vi "Subscribe to Results.vi"(8 "error in (no error)":errorcluster, 10 "Result Observer":refnum<class "Result Observer.lvclass">, 11 "LUnit Test Case V2 In":refnum<class "LUnit Test Case V2.lvclass">) -> (0 "error out":errorcluster, 3 "LUnit Test Case V2 Out":refnum<class "LUnit Test Case V2.lvclass">)   [LabVIEW 2020, in "LUnit Test Case V2.lvclass"]
uses:
  LUnit Test Case V2.lvclass
  Result Observer/Result Observer.lvclass
  LUnit Test Case V2.lvclass/LUnit Test Case V2.ctl
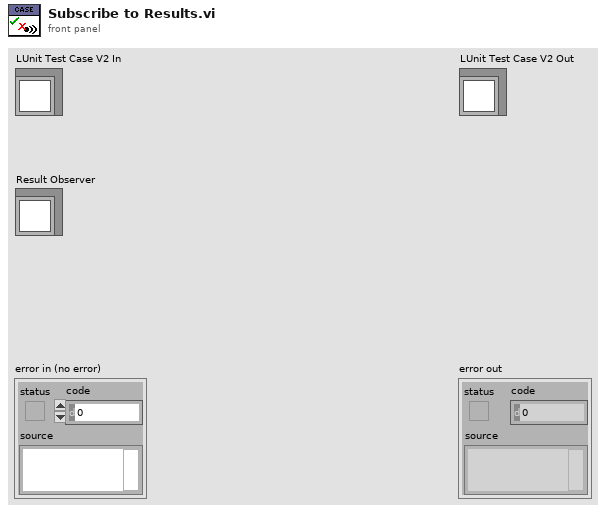
[diagram p1: front panel]
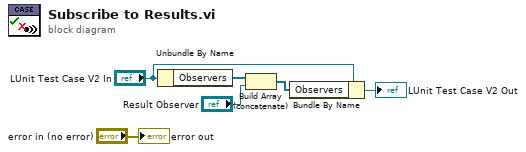
[diagram p0: block diagram]
diagram:
  n1 = Unbundle By Name("LUnit Test Case V2 In") -> ("Observers"=w4:refnum<class "Result Observer.lvclass">[])
  n2 = Build Array (concatenate)(w4, "Result Observer") -> (w2:refnum<class "Result Observer.lvclass">[])
  n3 = Bundle By Name(cluster="LUnit Test Case V2 In", "Observers"=w2) -> (→"LUnit Test Case V2 Out":refnum<class "LUnit Test Case V2.lvclass">)
  "error out" <- "error in (no error)"
